vi "MTMount_getNextSample_Cooling.vi"(8 "error in (no error)":errorcluster, 11 "Cooling_Ctl":T1) -> (0 "error out":errorcluster, 2 "function return":i32, 3 "Cooling_Ctl out":T1)   [LabVIEW 2018, in "SALLV_MTMount.lvlib"]
doc: "int MTMount_shm_getNextSample_CoolingLV(MTMount_CoolingLV *Cooling_Ctl );"
uses:
  SALLV_MTMount.lvlib
  DataTypes/Cooling.ctl
  SALLV_MTMount.so
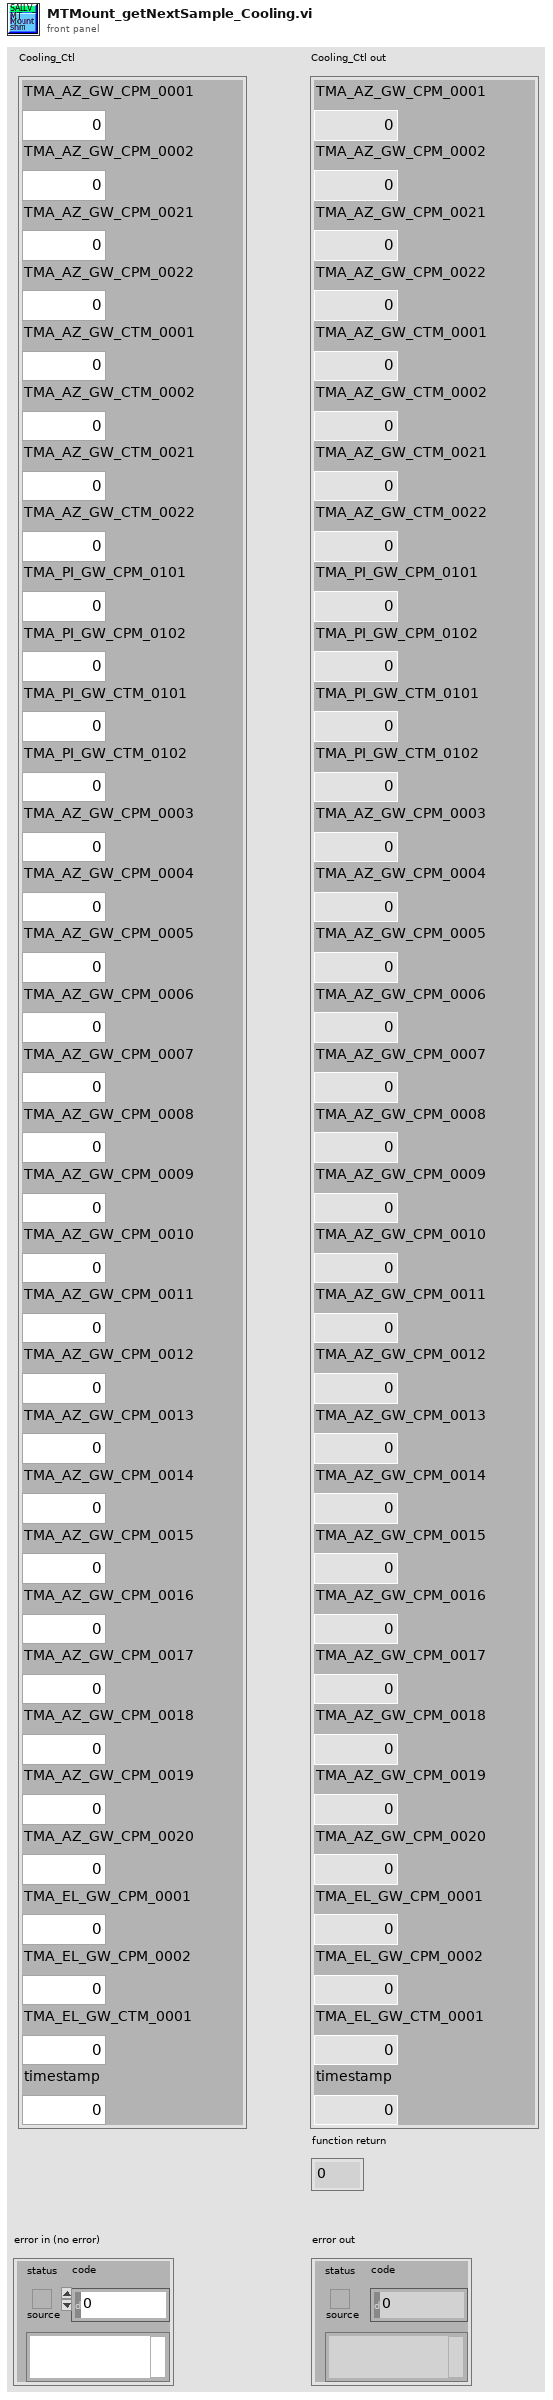
[diagram p1: front panel]
types:
  T1 = typedef "SALLV_MTMount.lvlib/Cooling.ctl" = cluster{"TMA_AZ_GW_CPM_0001":dbl, "TMA_AZ_GW_CPM_0002":dbl, "TMA_AZ_GW_CPM_0021":dbl, "TMA_AZ_GW_CPM_0022":dbl, "TMA_AZ_GW_CTM_0001":dbl, "TMA_AZ_GW_CTM_0002":dbl, "TMA_AZ_GW_CTM_0021":dbl, "TMA_AZ_GW_CTM_0022":dbl, "TMA_PI_GW_CPM_0101":dbl, "TMA_PI_GW_CPM_0102":dbl, "TMA_PI_GW_CTM_0101":dbl, "TMA_PI_GW_CTM_0102":dbl, "TMA_AZ_GW_CPM_0003":dbl, "TMA_AZ_GW_CPM_0004":dbl, "TMA_AZ_GW_CPM_0005":dbl, "TMA_AZ_GW_CPM_0006":dbl, "TMA_AZ_GW_CPM_0007":dbl, "TMA_AZ_GW_CPM_0008":dbl, "TMA_AZ_GW_CPM_0009":dbl, "TMA_AZ_GW_CPM_0010":dbl, "TMA_AZ_GW_CPM_0011":dbl, "TMA_AZ_GW_CPM_0012":dbl, "TMA_AZ_GW_CPM_0013":dbl, "TMA_AZ_GW_CPM_0014":dbl, "TMA_AZ_GW_CPM_0015":dbl, "TMA_AZ_GW_CPM_0016":dbl, "TMA_AZ_GW_CPM_0017":dbl, "TMA_AZ_GW_CPM_0018":dbl, "TMA_AZ_GW_CPM_0019":dbl, "TMA_AZ_GW_CPM_0020":dbl, "TMA_EL_GW_CPM_0001":dbl, "TMA_EL_GW_CPM_0002":dbl, "TMA_EL_GW_CTM_0001":dbl, "timestamp":dbl}
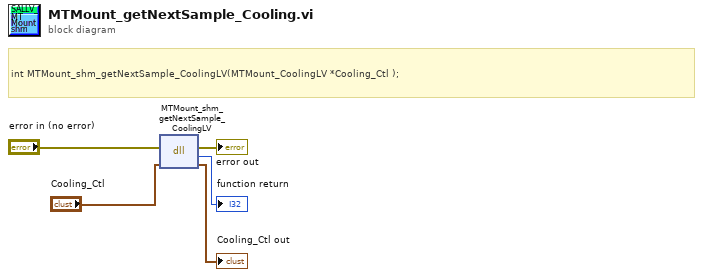
[diagram p0: block diagram]
diagram:
  # "int MTMount_shm_getNextSample_CoolingLV(MTMount_CoolingLV *Cooling_Ctl );"
  n1 = dll-call lib="home/ttsai/Document/salApiMTMount/SALLV_MTMount/SALLV_MTMount.*" fn="MTMount_shm_getNextSample_CoolingLV"(error in="error in (no error)", "Cooling_Ctl"="Cooling_Ctl") -> (error out=→"error out":errorcluster, →"function return":i32, "Cooling_Ctl"=→"Cooling_Ctl out":T1)  [unwired: 2 in, 1 out]
